vi "s3.vi"() -> ()   [LabVIEW 2020]
panel:
  in  "stop":bool
  out "XY Graph":cluster{"Y":dbl[], "Y":dbl[]}[](graph)
  out "build xy":dbl[](graph)
  out "Numeric":i32
  out "Waveform Graph":dynamicdata(graph)
  out "signle sample":dynamicdata(graph)
  in  "amptude":dbl
  in  "frequency":dbl
  in  "offset":dbl
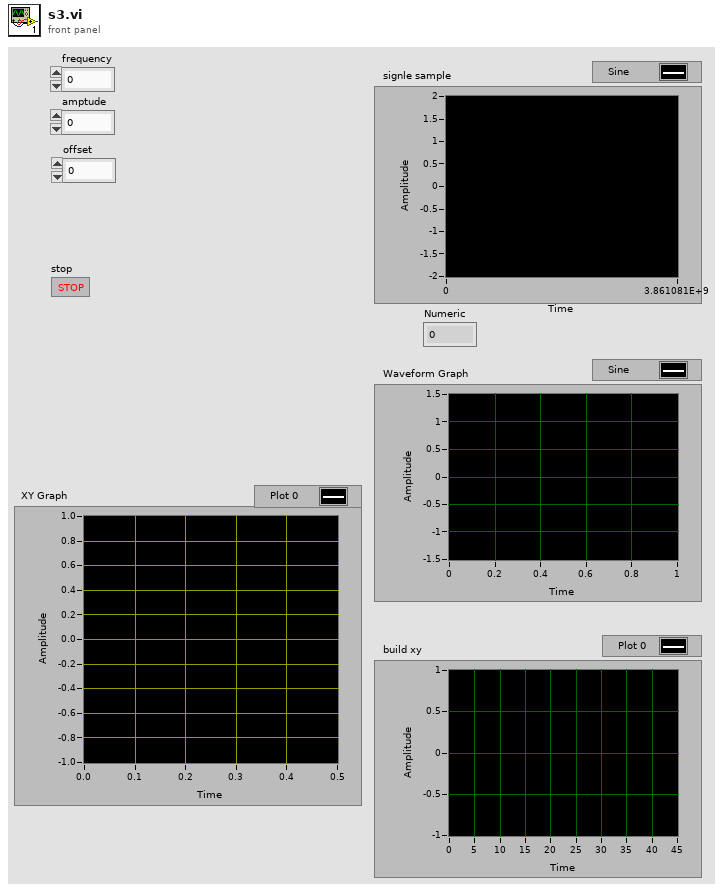
[diagram p1: front panel]
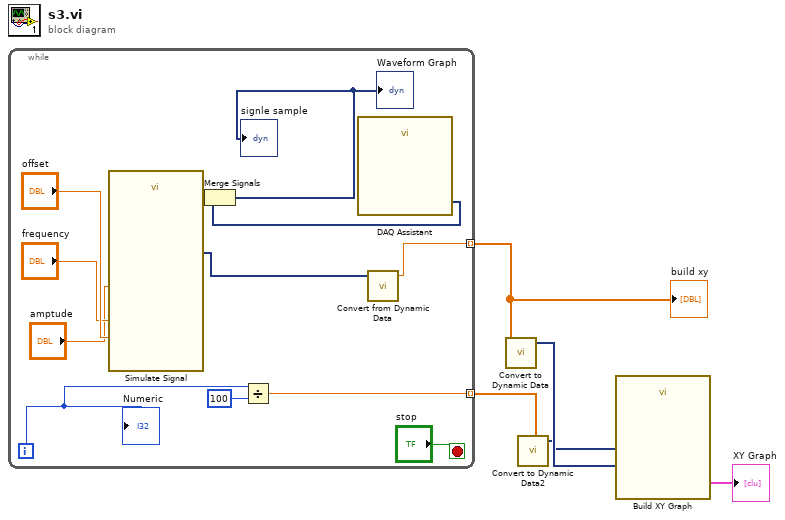
[diagram p0: block diagram]
diagram:
  n1 = while {
    tunnel: [w13] -> w3 mode=indexing
    tunnel: [w10] -> w5 mode=indexing
    i -> [w12]
    stop <- "stop" stop-if-true
    n2 = call "Simulate Signal"("Offset"="offset", "Frequency"="frequency", "Amplitude"="amptude") -> ("Sine"=w8:dynamicdata)  [unwired: 11 in, 1 out]
    n3 = Divide(x=w12, y=100) -> (x/y=w10:dbl)
    n4 = call "DAQ Assistant"() -> ("data"=w6:dynamicdata)  [unwired: 17 in, 2 out]
    n5 = Merge Signals(w8, w6) -> (→"signle sample" →"Waveform Graph":dynamicdata)
    n6 = call "Convert from Dynamic Data"("Dynamic Data Type"=w8) -> ("Scalar"=w13:dbl)  [unwired: 3 in]
    "Numeric" <- w12
  }
  "build xy" <- w3
  n7 = call "Convert to Dynamic Data"("Array"=w3) -> ("Dynamic Data Type"=w2:dynamicdata)  [unwired: 3 in]
  n8 = call "Convert to Dynamic Data2"("Array"=w5) -> ("Dynamic Data Type"=w1:dynamicdata)  [unwired: 3 in]
  n9 = call "Build XY Graph"("Y Input"=w2, "X Input"=w1) -> ("XY Graph"=→"XY Graph":cluster{"X":dbl[], "Y":dbl[]}[])  [unwired: 8 in, 1 out]
